vi "Empty_Visco.vi"(7 "Retain?":bool, 8 "ms":u32=5000, 10 "RPM":i32=300, 11 "Strokes":i32=350) -> ()   [LabVIEW 2019]
panel:
  out "Iterations":i32
  out "BlowOutIteration":i32
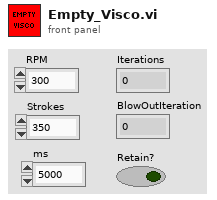
[diagram p1: front panel]
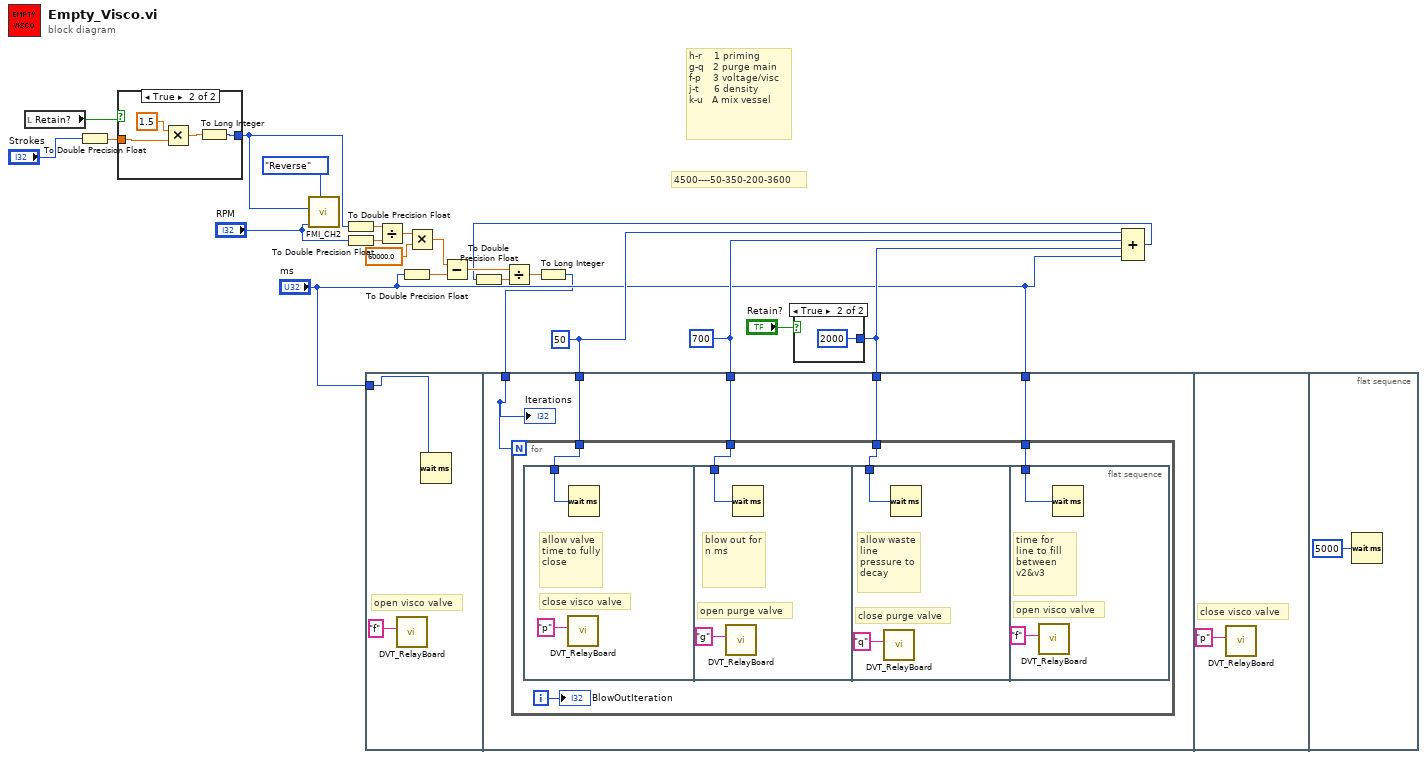
[diagram p0: block diagram]
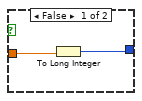
[diagram p2: hidden frame]
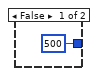
[diagram p3: hidden frame]
diagram:
  w17 = u32 700 ("milliseconds to wait")
  w16 = u32 50 ("milliseconds to wait")
  # "4500----50-350-200-3600"
  # "h-r    1 priming\ng-q   2 purge main\nf-p    3 voltage/visc\nj-t     6 density\nk-u   A mix vessel"
  n1 = local read "Retain?"() -> (w6:bool)
  n2 = To Double Precision Float(number="Strokes") -> (double precision float=w5:dbl)
  n3 = case shown="True" w6 {
    tunnel: w5 -> [w24 w28]
    tunnel: [w23 w25] -> w3
    frame False {
      n4 = To Long Integer(number=w24) -> (32bit integer=w23:i32)
    }
    frame True {
      n5 = Multiply(x=1.5, y=w28) -> (x*y=w26:dbl)
      n6 = To Long Integer(number=w26) -> (32bit integer=w25:i32)
    }
  }
  n7 = call "FMI_CH2.vi"("Direction"=enum16{"Forward", "Reverse"}."Reverse", "RPM"="RPM", "Strokes"=w3) -> ()  [unwired: 4 in, 1 out]
  n8 = To Double Precision Float(number=w3) -> (double precision float=w8:dbl)
  n9 = To Double Precision Float(number="RPM") -> (double precision float=w9:dbl)
  n10 = flat-sequence {
    tunnel: "ms" -> [w29]
    tunnel: "ms" -> [w35]
    tunnel: w18 -> [w34]
    tunnel: w17 -> [w33]
    tunnel: w16 -> [w32]
    tunnel: w1 -> [w31]
    frame #0 {
      # "open visco valve"
      n11 = call "DVT_RelayBoard.vi"("write buffer"="f") -> ()  [unwired: 3 in, 3 out]
      n12 = Wait (ms)(milliseconds to wait=w29) -> ()  [unwired: 1 out]
    }
    frame #1 {
      n13 = for {
        N: w31 -> [_]
        tunnel: w35 -> [w39]
        tunnel: w34 -> [w38]
        tunnel: w33 -> [w37]
        tunnel: w32 -> [w36]
        i -> [w40]
        n14 = flat-sequence {
          tunnel: w36 -> [w41]
          tunnel: w37 -> [w43]
          tunnel: w38 -> [w45]
          tunnel: w39 -> [w47]
          frame #0 {
            # "close visco valve"
            # "allow valve time to fully close"
            n15 = call "DVT_RelayBoard.vi"("write buffer"="p") -> ()  [unwired: 3 in, 3 out]
            n16 = Wait (ms)(milliseconds to wait=w41) -> ()  [unwired: 1 out]
          }
          frame #1 {
            # "open purge valve"
            # "blow out for n ms"
            n17 = call "DVT_RelayBoard.vi"("write buffer"="g") -> ()  [unwired: 3 in, 3 out]
            n18 = Wait (ms)(milliseconds to wait=w43) -> ()  [unwired: 1 out]
          }
          frame #2 {
            # "close purge valve"
            # "allow waste line pressure to decay"
            n19 = call "DVT_RelayBoard.vi"("write buffer"="q") -> ()  [unwired: 3 in, 3 out]
            n20 = Wait (ms)(milliseconds to wait=w45) -> ()  [unwired: 1 out]
          }
          frame #3 {
            # "open visco valve"
            # "time for line to fill between v2&v3"
            n21 = call "DVT_RelayBoard.vi"("write buffer"="f") -> ()  [unwired: 3 in, 3 out]
            n22 = Wait (ms)(milliseconds to wait=w47) -> ()  [unwired: 1 out]
          }
        }
        "BlowOutIteration" <- w40
      }
      "Iterations" <- w31
    }
    frame #2 {
      # "close visco valve"
      n23 = call "DVT_RelayBoard.vi"("write buffer"="p") -> ()  [unwired: 3 in, 3 out]
    }
    frame #3 {
      n24 = Wait (ms)(milliseconds to wait=u32 5000) -> ()  [unwired: 1 out]
    }
  }
  n25 = Divide(x=w8, y=w9) -> (x/y=w21:dbl)
  n26 = To Double Precision Float(number="ms") -> (double precision float=w11:dbl)
  n27 = Multiply(x=w21, y=60000.0 ("x/y")) -> (x*y=w19:dbl)
  n28 = Subtract(x=w19, y=w11) -> (x-y=w15:dbl)
  n29 = case shown="True" "Retain?" {
    tunnel: [u32 500 ("milliseconds to wait") u32 2000 ("milliseconds to wait")] -> w18
    frame False {
    }
    frame True {
    }
  }
  n30 = Compound Arithmetic op=ADD(w16, w17, w18, "ms") -> (w13:u32)
  n31 = To Double Precision Float(number=w13) -> (double precision float=w12:dbl)
  n32 = Divide(x=w15, y=w12) -> (x/y=w14:dbl)
  n33 = To Long Integer(number=w14) -> (32bit integer=w1:i32)
